vi "GetKeyType.vi"(8 "error in (no error)":errorcluster, 11 "Map in":refnum<class "Map.lvclass">) -> (0 "error out":errorcluster, 2 "Type":T1, 3 "Map out":refnum<class "Map.lvclass">)   [LabVIEW 2016, in "Map.lvclass"]
uses:
  <userlib>/836-libraries/Data_Structures/Map/Map.lvclass
  <vilib>/Utility/Data Type/Type Definitions/Data Type.ctl
  <userlib>/836-libraries/Data_Structures/Map/Map.lvclass/Map.ctl
  <vilib>/Utility/Data Type/NI_Data Type.lvlib
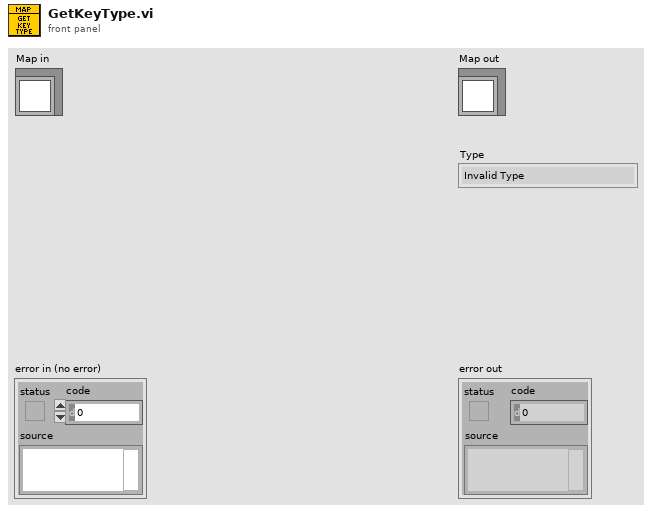
[diagram p1: front panel]
types:
  T1 = typedef "NI_Data Type.lvlib/Data Type.ctl" = enum8{"Invalid Type", "Void", "I8", "I16", "I32", "I64", "U8", "U16", "U32", "U64", "Single Float", "Double Float", "Extended Float", "Single Complex", "Double Complex", "Extended Complex", "Enum U8", "Enum U16", "Enum U32", "Enum U64", "Single Float With Unit", "Double Float With Unit", "Extended Float With Unit", "Single Complex with Unit", "Double Complex with Unit", "Extended Complex with Unit", "Boolean", "String", "Path", "Picture", "Tag", "Array", "Cluster", "Variant", "LV Variant", "Waveform", "Timestamp", "Digital Waveform", "Digital Data", "ExpressData", "Refnum", "External Data", "VI", "Poly VI", "LabVIEW Class Instance", "Fixed Point"}
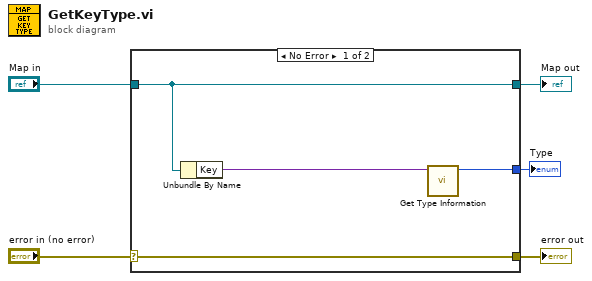
[diagram p0: block diagram]
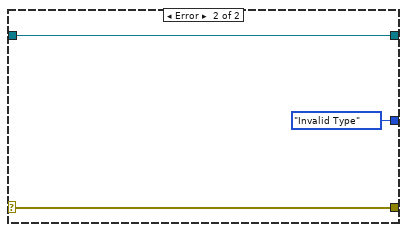
[diagram p2: hidden frame]
diagram:
  n1 = case shown="No Error" "error in (no error)" {
    selector: "error in (no error)" -> [w9 w11]
    tunnel: [w9 w11] -> w4
    tunnel: [w8 w12] -> w2
    tunnel: "Map in" -> [w8 w12]
    tunnel: [w6 Data_Type."Invalid Type" ("Type")] -> w1
    frame No Error {
      n2 = Unbundle By Name(w8) -> ("Key"=w7:variant)
      n3 = call <vilib>:"Get Type Information.vi"("Variant"=w7) -> ("Type"=w6:T1)  [unwired: 6 in, 4 out]
    }
    frame Error {
    }
  }
  "error out" <- w4
  "Map out" <- w2
  "Type" <- w1
